vi "Periodic Tasks.vi"(8 "error in":errorcluster) -> ()   [LabVIEW 2013]
doc: "This VI runs in parallel to other tasks. It can contain as many user-defined periodic loops as you need. These can carry out PID or other sorts of timed response."
uses:
  <vilib>/Rock Robotics/WPI/Joystick/WPI_JoystickButtonState.ctl
  <vilib>/Rock Robotics/SystemInterfaces/Utilities/FPGA_UtilitiesLED Source.ctl
  <vilib>/Rock Robotics/SystemInterfaces/Utilities/FPGA_UtilitiesLED State.ctl
  <vilib>/Rock Robotics/WPI/Compressor/WPI_CompressorGetSetRefNum.vi
  Robot Global Data.vi
  <vilib>/addons/control/pid/pid.llb/PID (DBL).vi
  <vilib>/Rock Robotics/WPI/RobotDrive/WPI_RobotDriveGetSetRefNum.vi
  <vilib>/Rock Robotics/WPI/Joystick/WPI_JoystickGetSetRefNum.vi
  <vilib>/addons/control/pid/NI_PID_pid.lvlib
panel:
  in  "Reset Zero Position":bool
  in  "Arm_Extend_Limit":dbl(slide)=4.0 scale=0.0..5.0
  in  "Arm_Retract_Limit":dbl(slide)=1.0 scale=0.0..5.0
  in  "ARM_HOME":dbl(slide)=0.53 scale=1.0..-1.0
  in  "Feeder_Arm_Speed":dbl
  out "JS1_BTNS":T1
  in  "Counter":i32
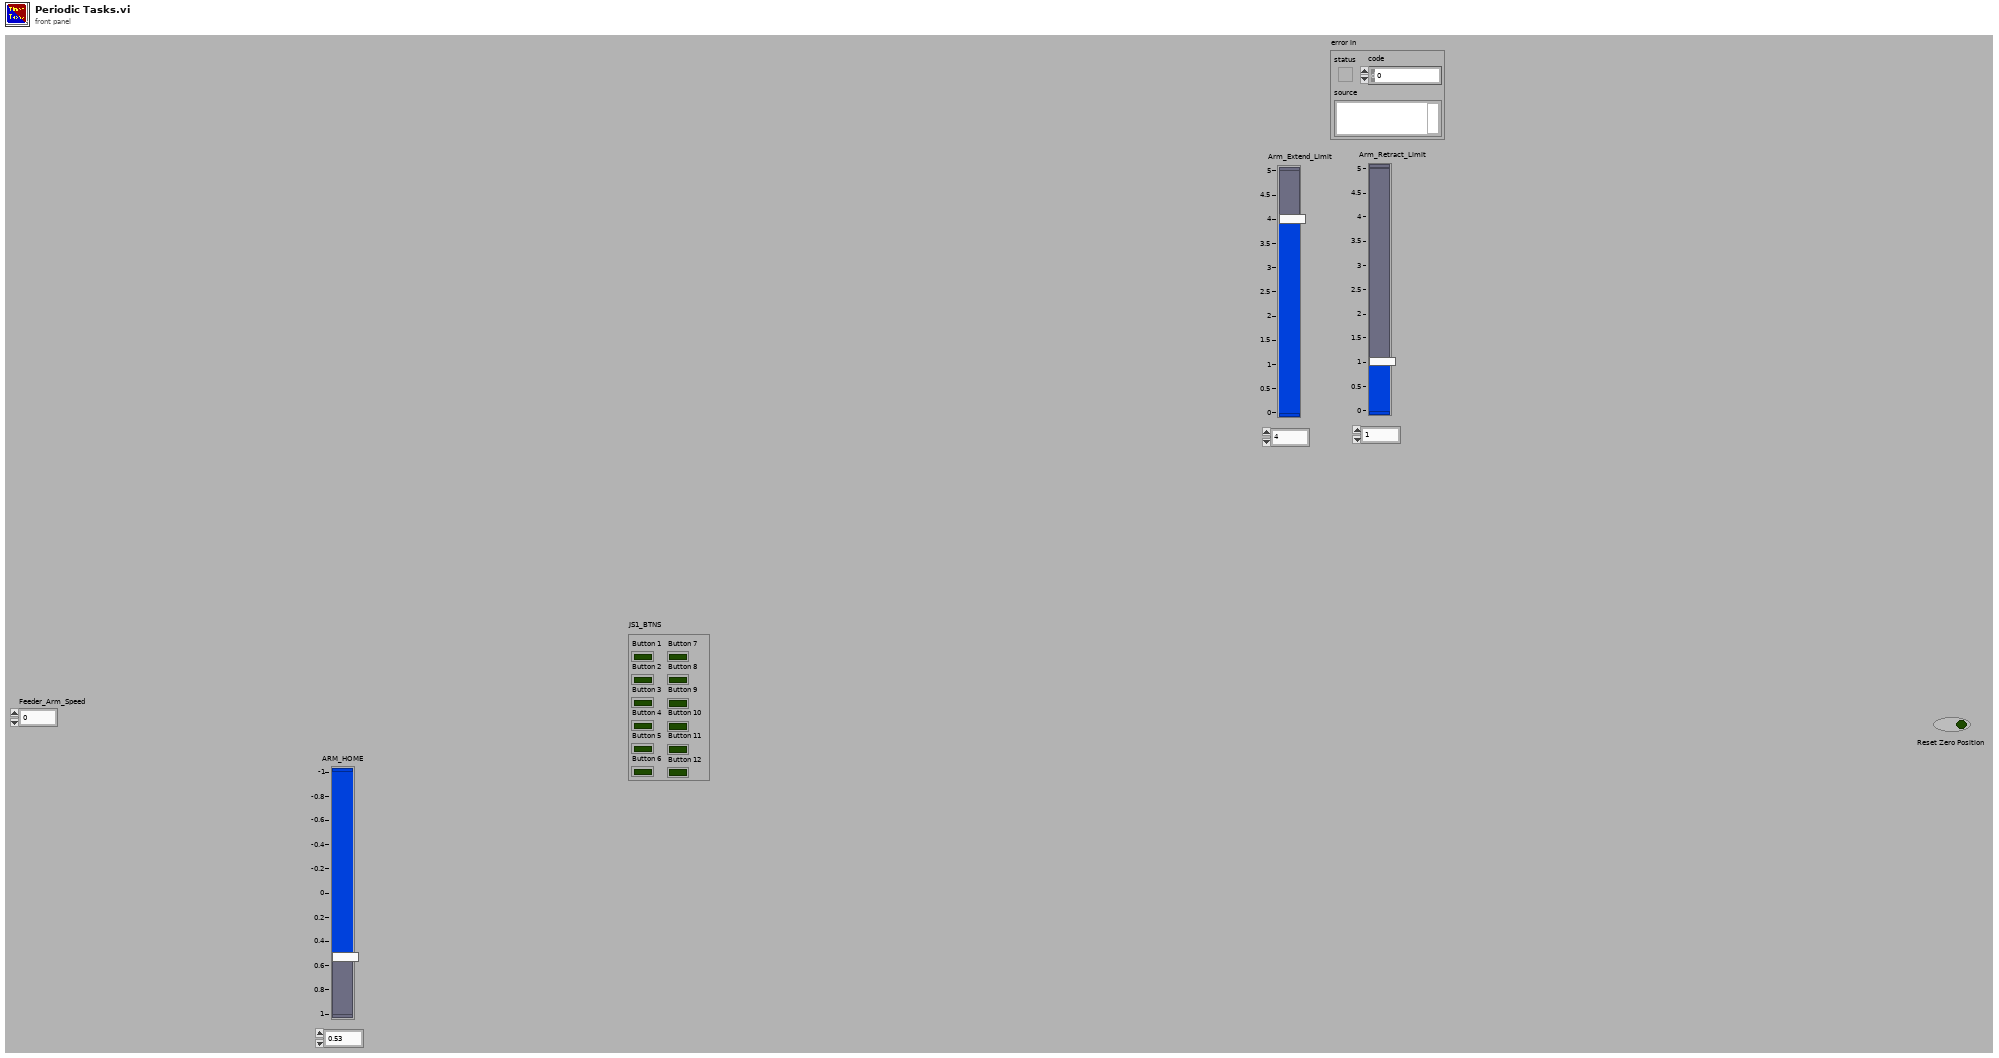
[diagram p1: front panel]
types:
  T1 = typedef "WPI_JoystickButtonState.ctl" = cluster{"Button 1":bool, "Button 2":bool, "Button 3":bool, "Button 4":bool, "Button 5":bool, "Button 6":bool, "Button 7":bool, "Button 8":bool, "Button 9":bool, "Button 10":bool, "Button 11":bool, "Button 12":bool}
  T2 = typedef "WPI_JoystickDevRef.ctl" = cluster{"Device":T3}
  T3 = typedef "WPI_JoystickDeviceEnum.ctl" = enum16{"USB 1", "USB 2", "USB 3", "USB 4", "Kinect 1", "Kinect 2"}
  T4 = typedef "WPI_RobotDriveDevRef.ctl" = cluster{"DevStatus":errorcluster, "Motors[]":T5[], "Square Inputs":bool, "Max Output":dbl, "Isochronous":bool}
  T5 = typedef "WPI_MotorControlDeviceRef.ctl" = cluster{"DeviceStatus":errorcluster, "Type":enum16{"PWM", "CAN"}, "PWM":cluster{"Digital Module":T6, "PWM Channel":T7, "DeadBand":T8}, "CAN":cluster{"Device Number":u8, "Control Mode":T9, "Semaphore":T10, "Max Vout":dbl}, "Invert":bool, "TransformRef":T11, "InvTransformRef":T11}
  T6 = typedef "FPGA_TypedefDigitalModule.ctl" = enum16{"Digital Module 1", "Digital Module 2"}
  T7 = typedef "FPGA_DIOPWMChannel.ctl" = enum8{"PWM 1", "PWM 2", "PWM 3", "PWM 4", "PWM 5", "PWM 6", "PWM 7", "PWM 8", "PWM 9", "PWM 10", "Invalid"}
  T8 = typedef "WPI_PWMDeadband.ctl" = cluster{"Name":string, "maxPositivePwm":i32, "minPositivePwm":i32, "centerPwm":i32, "maxNegativePwm":i32, "minNegativePwm":i32, "angularRange":u16}
  T9 = typedef "WPI_CANJaguar_ControlMode.ctl" = enum8{"Percent VBus", "Current", "Speed", "Position", "Voltage"}
  T10 = typedef "Semaphore RefNum" = refnum<k1>
  T11 = typedef "WPI_PWMTransform_ConPane.ctl" = refnum<vi>
  T12 = cluster{"JoystickDevRef":T2, "RobotDriveDevRef":T4}
  T13 = typedef "FPGA_UtilitiesLED State.ctl" = enum16{"Off", "On", "Toggle"}
  T14 = typedef "FPGA_UtilitiesLED Source.ctl" = enum16{"User LED", "FPGA LED"}
  T15 = typedef "WPI_CompressorDevRef.ctl" = cluster{"DevStatus":errorcluster, "DigitalInputDevRef":T16, "RelayDevRef":T18}
  T16 = typedef "WPI_DigitalInputDevRef.ctl" = cluster{"DevStatus":errorcluster, "DIO Channel":T17, "Digital Module":T6}
  T17 = typedef "FPGA_DIOChannel.ctl" = enum8{"DIO 1", "DIO 2", "DIO 3", "DIO 4", "DIO 5", "DIO 6", "DIO 7", "DIO 8", "DIO 9", "DIO 10", "DIO 11", "DIO 12", "DIO 13", "DIO 14", "Invalid"}
  T18 = typedef "WPI_RelayDevRef.ctl" = cluster{"DevStatus":errorcluster, "Relay Channel":T19, "Digital Module":T6, "Relay Direction":T20}
  T19 = typedef "FPGA_DIORelayChannel.ctl" = enum8{"Relay 1", "Relay 2", "Relay 3", "Relay 4", "Relay 5", "Relay 6", "Relay 7", "Relay 8", "Invalid"}
  T20 = typedef "WPI_RelayDirection.ctl" = enum16{"Both directions", "Forward only", "Reverse only"}
  T21 = typedef "WPI_AnalogChannelDevRef.ctl" = cluster{"DevStatus":errorcluster, "Analog Module":T22, "Analog Channel":T23}
  T22 = typedef "FPGA_TypedefAnalogModule.ctl" = enum16{"Analog Module 1", "Analog Module 2"}
  T23 = typedef "FPGA_AIChannel.ctl" = enum8{"AI 1", "AI 2", "AI 3", "AI 4", "AI 5", "AI 6", "AI 7", "AI 8", "Invalid"}
  T24 = typedef "WPI_GyroDevRef.ctl" = cluster{"DevStatus":errorcluster, "Analog Module":T22, "Analog Channel":T23, "Offset":dbl, "Gain (VoltsPerDegree/Second)":dbl}
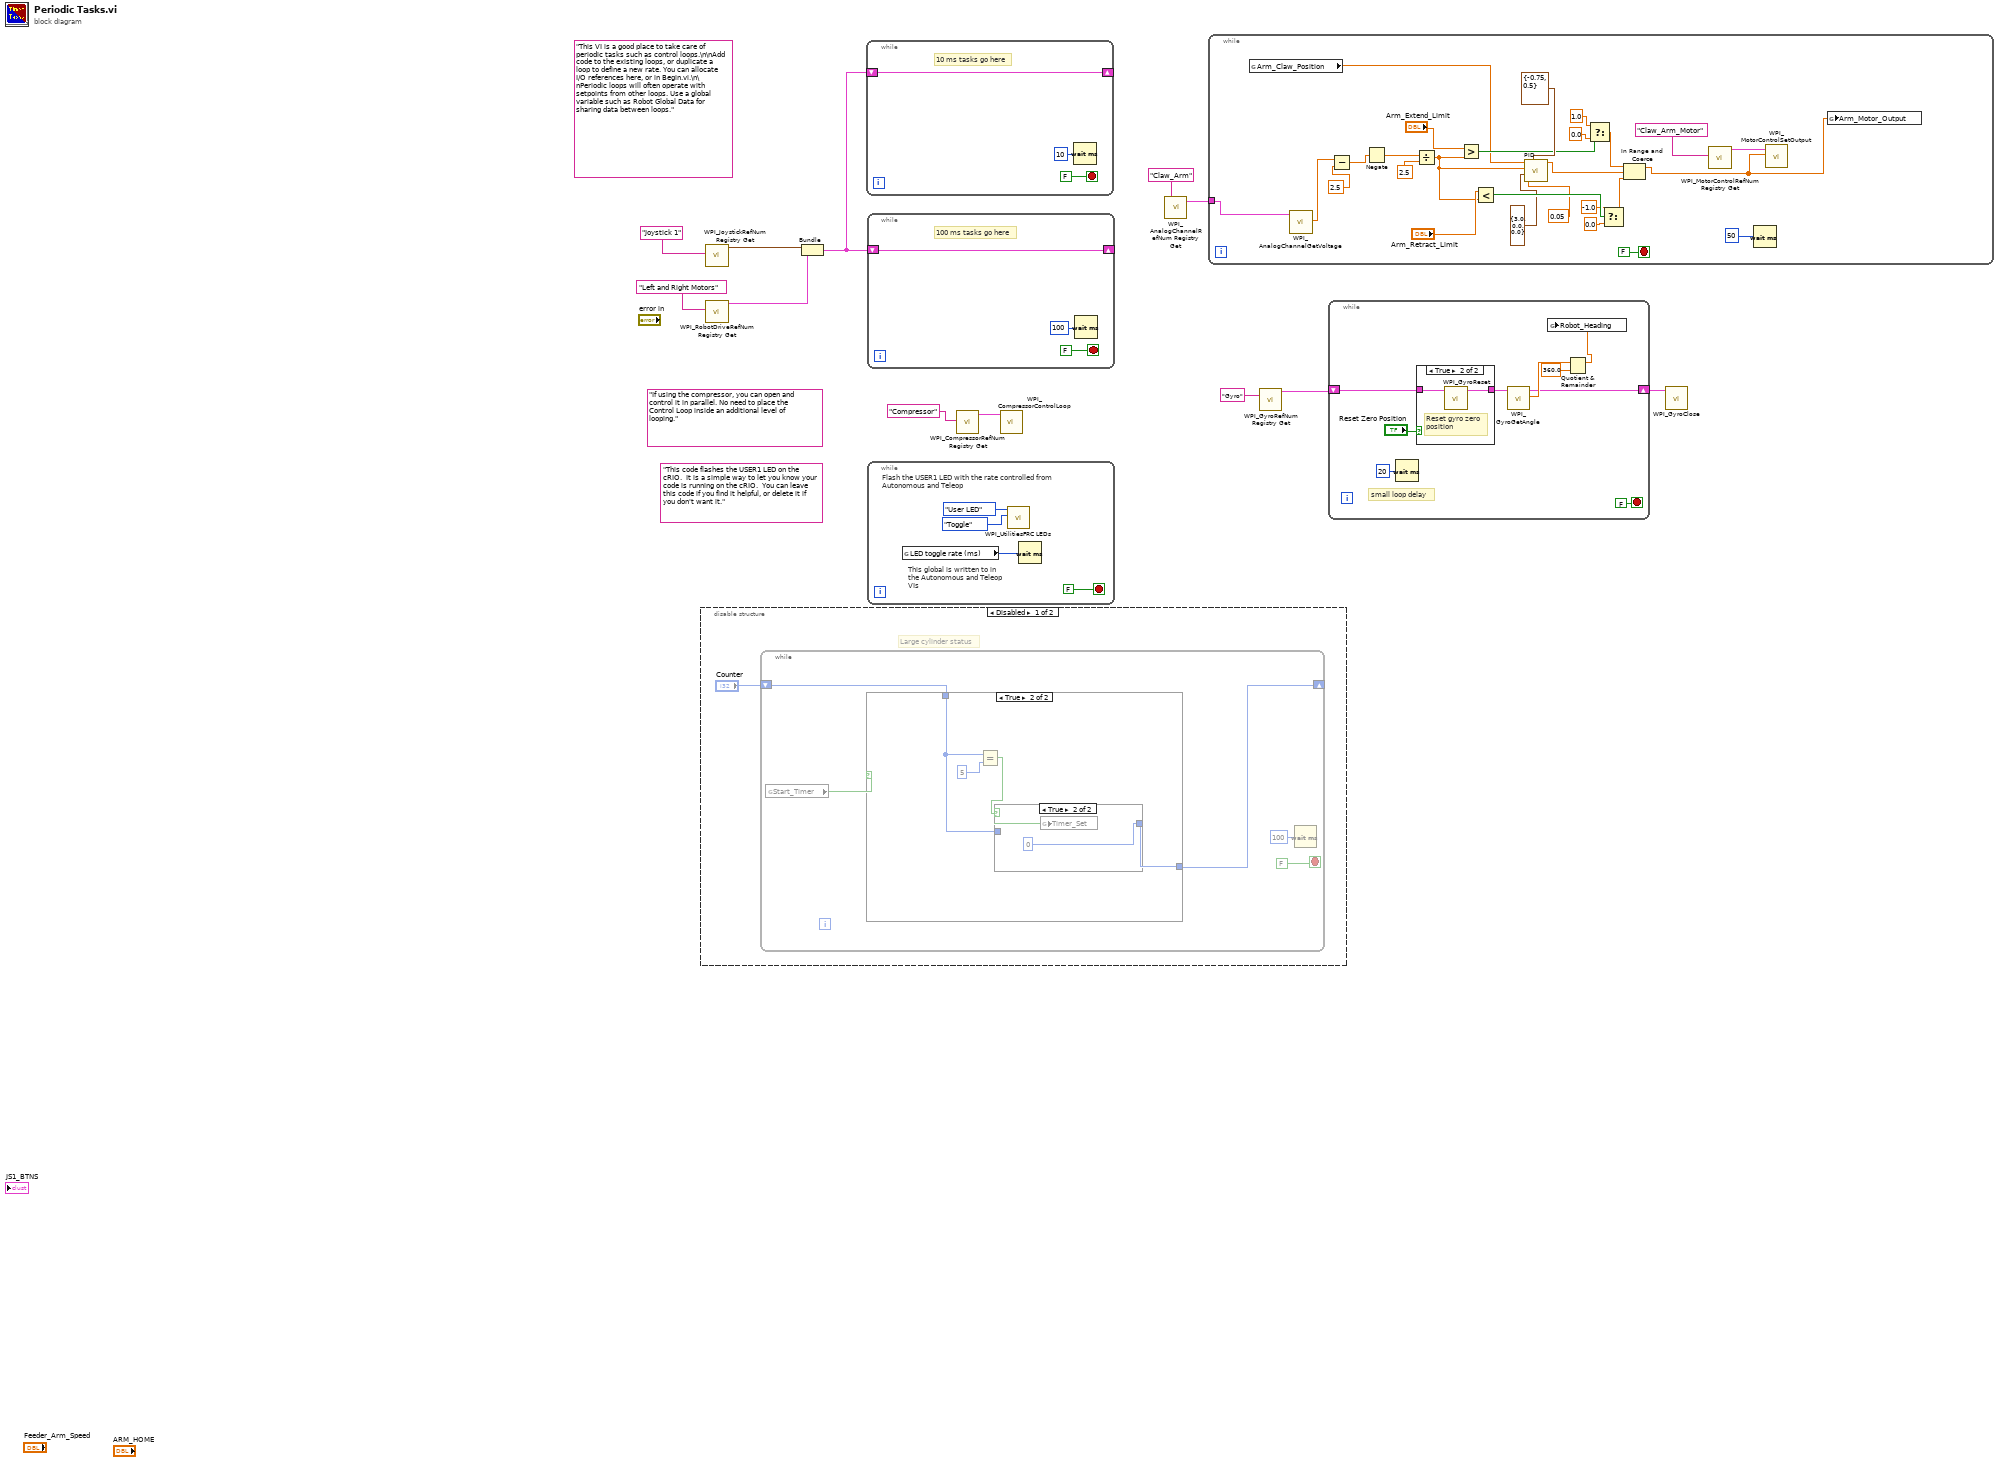
[diagram p0: block diagram]
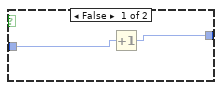
[diagram p4: hidden frame]
diagram:
  (unwired) "If using the compressor, you can open and control it in parallel. No need to place the Control Loop inside an additional level of looping."
  (unwired) "This code flashes the USER1 LED on the cRIO.  It is a simple way to let you know your code is running on the cRIO.  You can leave this code if you find it helpful, or delete it if you don't want it."
  (unwired) "This VI is a good place to take care of periodic tasks such as control loops.\n\nAdd code to the existing loops, or duplicate a loop to define a new rate. You can allocate I/O references here, or in Begin.vi.\n\nPeriodic loops will often operate with setpoints from other loops. Use a global variable such as Robot Global Data for sharing data between loops."
  n1 = disable-structure shown="Disabled" {
    frame Disabled {
      # "Large cylinder status"
      n2 = while {
        shift-right: [w14] -> _
        shift-left: "Counter" -> [w15]
        stop <- FALSE stop-if-true
        n3 = global read "Robot Global Data.vi" "Start_Timer"() -> (w16:bool)
        n4 = case shown="True" w16 {
          tunnel: w15 -> [w19 w23]
          tunnel: [w19 w22] -> w14
          frame False {
          }
          frame True {
            n5 = Equal?(x=w23, y=5) -> (x = y?=w20:bool)
            n6 = case shown="True" w20 {
              selector: w20 -> [_ w27]
              tunnel: [w25 0] -> w22
              tunnel: w23 -> [w24 _]
              frame False {
                n7 = Increment(x=w24) -> (x+1=w25:i32)
              }
              frame True {
                n8 = global write "Robot Global Data.vi" "Timer_Set"(w27) -> ()
              }
            }
          }
        }
        n9 = Wait (ms)(milliseconds to wait=u32 100) -> ()  [unwired: 1 out]
      }
    }
    frame Enabled {
    }
  }
  n10 = call <vilib>:"WPI_JoystickRefNum Registry Get.vi"("refnum name"="Joystick 1") -> ("JoystickDevRef"=w10:T2)  [unwired: 1 in, 9 out]
  n11 = call <vilib>:"WPI_RobotDriveRefNum Registry Get.vi"("refnum name"="Left and Right Motors") -> ("RobotDriveDevRef"=w9:T4)  [unwired: 1 in, 9 out]
  n12 = Bundle("JoystickDevRef"=w10, "RobotDriveDevRef"=w9) -> (w8:T12)  [unwired: 1 out]
  n13 = while {
    shift-right: [w28] -> _
    shift-left: w8 -> [w28]
    stop <- FALSE stop-if-true
    # "10 ms tasks go here"
    n14 = Wait (ms)(milliseconds to wait=u32 10) -> ()  [unwired: 1 out]
  }
  n15 = while {
    shift-right: [w31] -> _
    shift-left: w8 -> [w31]
    stop <- FALSE stop-if-true
    # "100 ms tasks go here"
    n16 = Wait (ms)(milliseconds to wait=u32 100) -> ()  [unwired: 1 out]
  }
  n17 = while {
    stop <- FALSE stop-if-true
    # "This global is written to in the Autonomous and Teleop VIs"
    # "Flash the USER1 LED with the rate controlled from Autonomous and Teleop"
    n18 = global read "Robot Global Data.vi" "LED toggle rate (ms)"() -> (w34:u32)
    n19 = call <vilib>:"WPI_UtilitiesFRC LEDs.vi"("State"=FPGA_UtilitiesLED_State."Toggle", "LED Type"=FPGA_UtilitiesLED_Source."User LED") -> ()  [unwired: 1 in, 9 out]
    n20 = Wait (ms)(milliseconds to wait=w34) -> ()  [unwired: 1 out]
  }
  n21 = call <vilib>:"WPI_CompressorRefNum Registry Get.vi"("refnum name"="Compressor") -> ("CompressorDevRef"=w6:T15)  [unwired: 9 in, 1 out]
  n22 = call <vilib>:"WPI_CompressorControlLoop.vi"("CompressorDevRef"=w6) -> ()  [unwired: 11 in]
  n23 = call <vilib>:"WPI_AnalogChannelRefNum Registry Get.vi"("refnum name"="Claw_Arm") -> ("AIDeviceRef"=w1:T21)  [unwired: 1 in, 9 out]
  n24 = while {
    tunnel: w1 -> [w38]
    stop <- FALSE stop-if-true
    n25 = global read "Robot Global Data.vi" "Arm_Claw_Position"() -> (w45:dbl)
    n26 = call <vilib>:"WPI_AnalogChannelGetVoltage.vi"("AIDeviceRef"=w38) -> ("Voltage"=w47:dbl)  [unwired: 1 in, 9 out]
    n27 = Subtract(x=w47, y=2.5) -> (x-y=w50:dbl)
    n28 = Negate(x=w50) -> (-x=w51:dbl)
    n29 = Divide(x=w51, y=2.5) -> (x/y=w48:dbl)
    n30 = Greater?(x="Arm_Extend_Limit", y=w48) -> (0:w59:bool)
    n31 = Less?(x="Arm_Retract_Limit", y=w48) -> (x < y?=w61:bool)
    n32 = call-poly <vilib>:"PID.vi"("output range"=cluster{"output low":dbl, "output high":dbl} {"output low"=-0.75, "output high"=0.5}, "dt (s)"=0.05, "PID gains"=cluster{dbl, dbl, dbl} {3.0, 0.0, 0.0}, "process variable"=w48, "setpoint"=w45) -> ("output"=w52:dbl)  [unwired: 1 in, 5 out]
    n33 = Select(t=1.0, s=w59, f=0.0) -> (s? t:f=w57:dbl)
    n34 = Select(t=-1.0, s=w61, f=0.0) -> (s? t:f=w58:dbl)
    n35 = In Range and Coerce(upper limit=w57, x=w52, lower limit=w58) -> (coerced(x)=w39:dbl)  [unwired: 1 out]
    n36 = call <vilib>:"WPI_MotorControlRefNum Registry Get.vi"("refnum name"="Claw_Arm_Motor") -> ("MotorControlDevRef"=w41:T5)  [unwired: 1 in, 9 out]
    n37 = Wait (ms)(milliseconds to wait=50) -> ()  [unwired: 1 out]
    n38 = call <vilib>:"WPI_MotorControlSetOutput.vi"("Output"=w39, "MotorControlDevRef"=w41) -> ()  [unwired: 3 in, 7 out]
    n39 = global write "Robot Global Data.vi" "Arm_Motor_Output"(w39) -> ()
  }
  n40 = call <vilib>:"WPI_GyroRefNum Registry Get.vi"("refnum name"="Gyro") -> ("GyroDevRef"=w3:T24)  [unwired: 9 in, 1 out]
  n41 = while {
    shift-right: [w69] -> w5
    shift-left: w3 -> [w72]
    stop <- FALSE stop-if-true
    # "small loop delay"
    n42 = Wait (ms)(milliseconds to wait=u32 20) -> ()  [unwired: 1 out]
    n43 = case shown="True" "Reset Zero Position" {
      tunnel: w72 -> [w74 w76]
      tunnel: [w74 w75] -> w71
      frame False {
      }
      frame True {
        # "Reset gyro zero \nposition"
        n44 = call <vilib>:"WPI_GyroReset.vi"("GyroDevRef"=w76) -> ("GyroDevRef"=w75:T24)  [unwired: 10 out]
      }
    }
    n45 = call <vilib>:"WPI_GyroGetAngle.vi"("GyroDevRef"=w71) -> ("Angle"=w70:dbl, "GyroDevRef"=w69:T24)  [unwired: 1 in, 8 out]
    n46 = Quotient & Remainder(x=w70, y=360.0) -> (x-y*floor(x/y)=w65:dbl)  [unwired: 1 out]
    n47 = global write "Robot Global Data.vi" "Robot_Heading"(w65) -> ()
  }
  n48 = call <vilib>:"WPI_GyroClose.vi"("GyroDevRef"=w5) -> ()  [unwired: 1 in, 10 out]
